vi "ReadImage.vi"() -> ()   [LabVIEW 2014]
panel:
  in  "ImgTypeSet":T1 items=["Grayscale (U8)", "Grayscale (I16)", "Grayscale (SGL)", "Complex (CSG)", "RGB (U32)", "HSL (U32)", "RGB (U64)", "Grayscale (U16)"]
  out "ImageTypeGet":T1 items=["Grayscale (U8)", "Grayscale (I16)", "Grayscale (SGL)", "Complex (CSG)", "RGB (U32)", "HSL (U32)", "RGB (U64)", "Grayscale (U16)"]
  out "Image":T2(plugin-control)
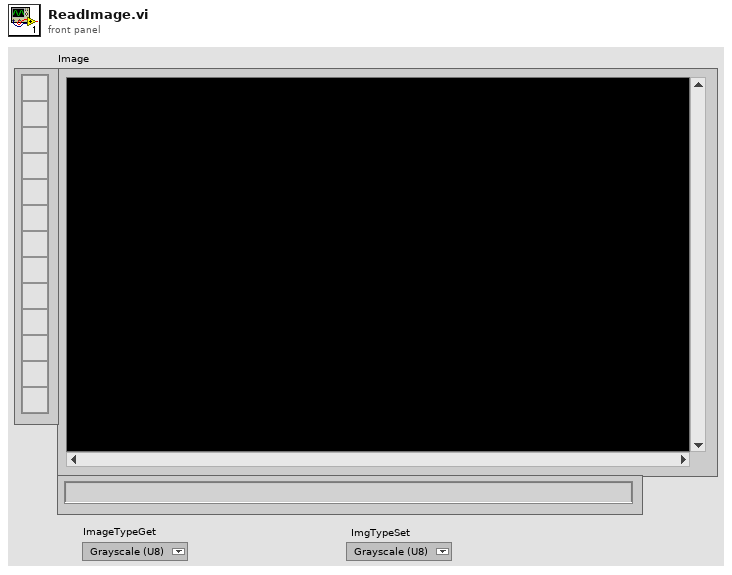
[diagram p1: front panel]
types:
  T1 = typedef "Image Type" = u32
  T2 = typedef "IMAQ Image.ctl" = refnum<image>
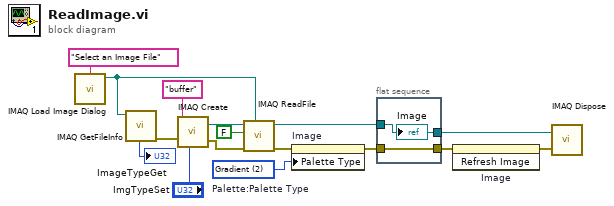
[diagram p0: block diagram]
diagram:
  w5 = u32 2 items=["Grayscale", "Binary", "Gradient", "Rainbow", "Temperature", "User Defined"]  # Palette:Palette Type
  n1 = call "IMAQ Load Image Dialog"("Prompt"="Select an Image File" ("prompt")) -> ("Path"=w10:path)  [unwired: 8 in, 2 out]
  n2 = call "IMAQ GetFileInfo"("File Path"=w10) -> ("error out"=w9:errorcluster, "Image Type"=→"ImageTypeGet":T1)  [unwired: 4 in, 5 out]
  n3 = call "IMAQ Create"("Image Name"="buffer", "Image Type"="ImgTypeSet", "error in (no error)"=w9) -> ("New Image"=w15:T2, "error out"=w14:errorcluster)  [unwired: 2 in]
  n4 = call "IMAQ ReadFile"("File Path"=w10, "error in (no error)"=w14, "Load Color Palette? (No)"=FALSE, "Image"=w15) -> ("error out"=w4:errorcluster, "Image Out"=w13:T2)  [unwired: 3 in, 3 out]
  n5 = property on="Image" class="ImageControl"(error in=w4, "Palette Type"=w5) -> (error out=w3:errorcluster)  [unwired: 1 in, 1 out]
  n6 = flat-sequence {
    tunnel: w13 -> [w17]
    tunnel: [w18] -> w2
    tunnel: w3 -> [w18]
    tunnel: [w17] -> w12
    frame #0 {
      "Image" <- w17
    }
  }
  n7 = invoke on="Image" class="ImageControl" method="Refresh Image"(error in=w2) -> (error out=w1:errorcluster)  [unwired: 2 in, 2 out]
  n8 = call "IMAQ Dispose"("Image"=w12, "error in (no error)"=w1) -> ()  [unwired: 4 in, 1 out]
